vi "WebServer-BaseURL.vi"() -> (0 "Web Server:Active":bool, 1 "Web-Server:Base-URL":string)   [LabVIEW 2016, in "CS++Utilities.lvlib"]
doc: "This VI returns the local LabVIEW Web-Server Base-URL."
uses:
  CS++Utilities.lvlib
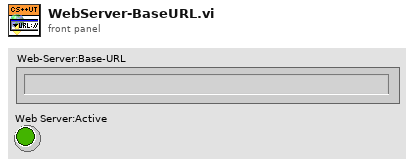
[diagram p1: front panel]
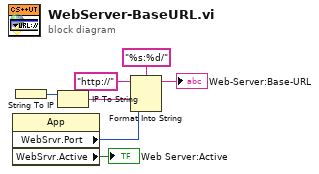
[diagram p0: block diagram]
diagram:
  n1 = property class="App"() -> ("WebSrvr.Port"=w6:u16, "WebSrvr.Active"=→"Web Server:Active":bool)  [unwired: 2 in, 2 out]
  n2 = String To IP() -> (0:w2:u32)  [unwired: 1 in]
  n3 = IP To String(2:w2) -> (0:w5:string)  [unwired: 1 in]
  n4 = Format Into String(format string="%s:%d/", initial string="http://" ("string"), w5, w6) -> (resulting string=→"Web-Server:Base-URL":string)  [unwired: 1 in, 1 out]
